vi "STOP_ALL.vi"(10 "argv":string[](array[string]), 11 "args":u8) -> ()   [LabVIEW 2015]
uses:
  Team Code/Robot Global Data.vi
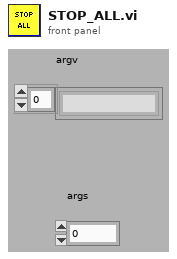
[diagram p1: front panel]
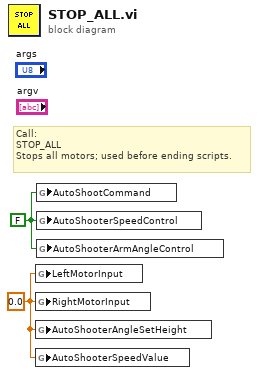
[diagram p0: block diagram]
diagram:
  w1 = FALSE ("AutoShooterSpeedControl")
  w2 = 0.0 ("RightMotorValue")
  # "Call:\nSTOP_ALL\nStops all motors; used before ending scripts."
  n1 = global write "Robot Global Data.vi" "LeftMotorInput"(w2) -> ()
  n2 = global write "Robot Global Data.vi" "RightMotorInput"(w2) -> ()
  n3 = global write "Robot Global Data.vi" "AutoShooterAngleSetHeight"(w2) -> ()
  n4 = global write "Robot Global Data.vi" "AutoShooterSpeedValue"(w2) -> ()
  n5 = global write "Robot Global Data.vi" "AutoShootCommand"(w1) -> ()
  n6 = global write "Robot Global Data.vi" "AutoShooterSpeedControl"(w1) -> ()
  n7 = global write "Robot Global Data.vi" "AutoShooterArmAngleControl"(w1) -> ()
